vi "Get Worker Terminals.vi"(11 "Worker VI":refnum<vi>) -> (1 "Special Terminals":T1, 2 "Types":T2[](array[typedef]), 3 "Worker VI out":refnum<vi>)   [LabVIEW 2020, in "FlexBlock.xnode"]
uses:
  FlexBlock.xnode
  FlexBlocks/Type Descriptor.ctl
  FlexBlocks/Terminal Direction.ctl
  FlexBlocks/Value Mode.ctl
  FlexBlocks/Terminal State.ctl
  FlexBlocks/Special Terminal.ctl
  FlexBlocks/Special Terminal Indices.ctl
  FlexBlocks/Worker Action.ctl
  FlexBlocks/FlexBlocks.lvlib
  <vilib>/Utility/Data Type/NI_Data Type.lvlib
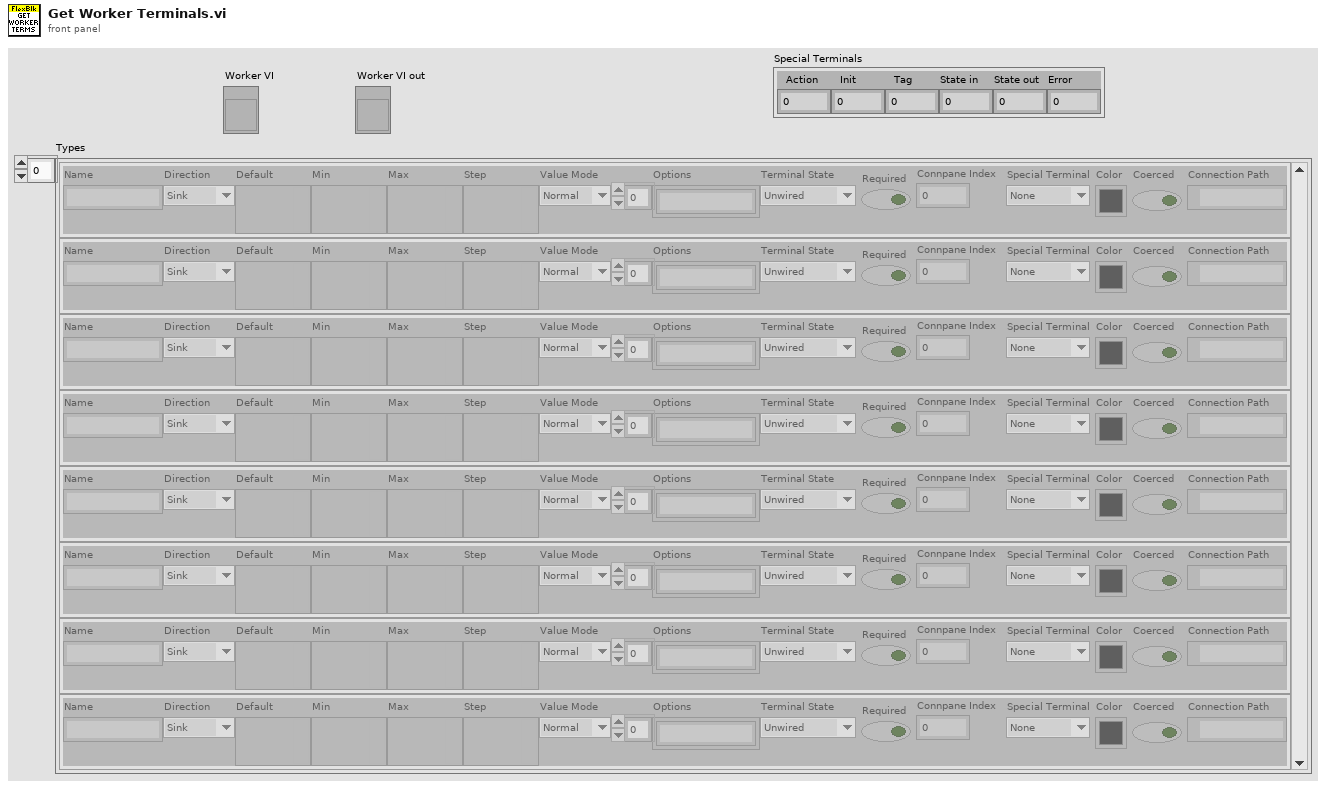
[diagram p1: front panel]
types:
  T1 = typedef "FlexBlocks.lvlib/Special Terminal Indices.ctl" = cluster{"Action":i32, "Init":i32, "Tag":i32, "State in":i32, "State out":i32, "Error":i32}
  T2 = typedef "FlexBlocks.lvlib/Type Descriptor.ctl" = cluster{"Name":string, "Direction":T3, "Default":variant, "Min":variant, "Max":variant, "Step":variant, "Value Mode":T4, "Options":string[], "Terminal State":T5, "Required":bool, "Connpane Index":i32, "Special Terminal":T6, "Color":u32, "Coerced":bool, "Connection Path":path}
  T3 = typedef "FlexBlocks.lvlib/Terminal Direction.ctl" = enum16{"Sink", "Source"}
  T4 = typedef "FlexBlocks.lvlib/Value Mode.ctl" = enum16{"Normal", "Range", "Select"}
  T5 = typedef "FlexBlocks.lvlib/Terminal State.ctl" = enum16{"Unwired", "BadType", "BadRef", "Channel", "Value", "Control Ref"}
  T6 = typedef "FlexBlocks.lvlib/Special Terminal.ctl" = enum16{"None", "Action", "Init", "Tag", "State in", "State out", "Error"}
  T7 = typedef "FlexBlocks.lvlib/Worker Action.ctl" = enum16{"Start", "Work", "Stop"}
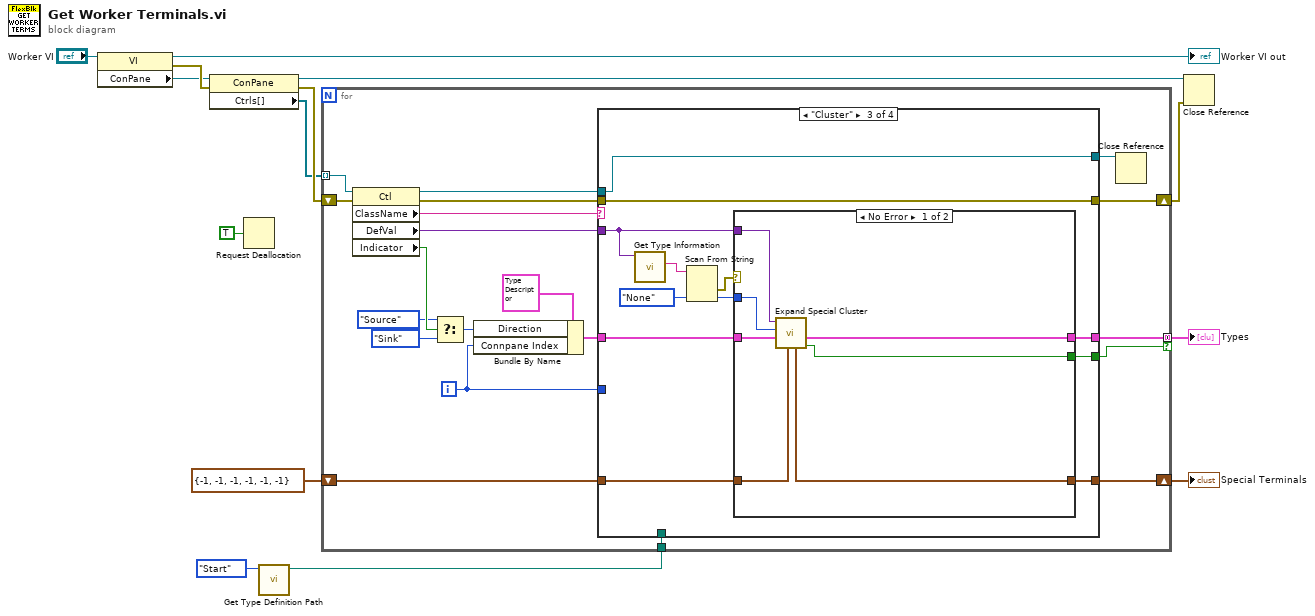
[diagram p0: block diagram]
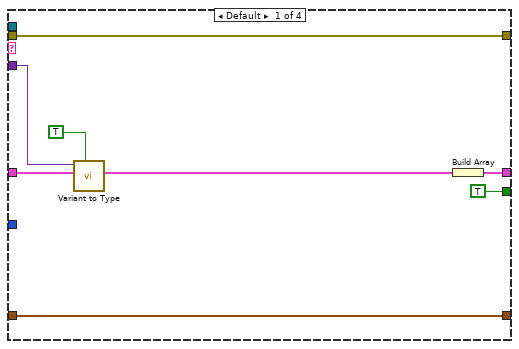
[diagram p2: hidden frame]
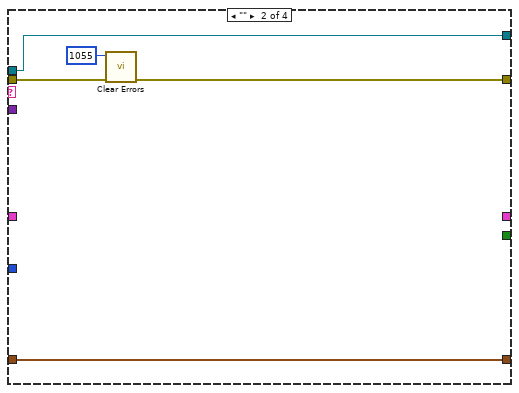
[diagram p3: hidden frame]
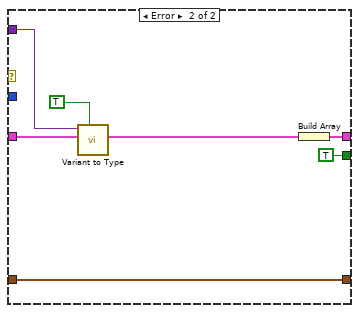
[diagram p4: hidden frame]
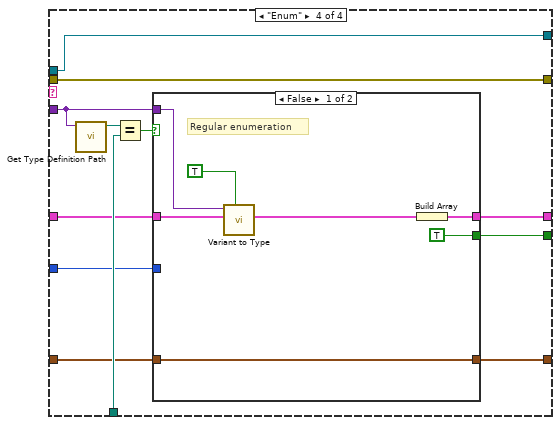
[diagram p5: hidden frame]
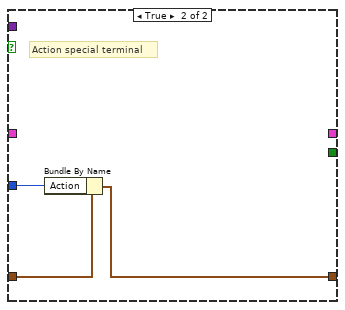
[diagram p6: hidden frame]
diagram:
  n1 = property class="VI"(reference="Worker VI") -> (reference out=→"Worker VI out":refnum<vi>, error out=w13:errorcluster, "ConPane"=w12:refnum<vi>)  [unwired: 1 in]
  n2 = property class="ConPane"(reference=w12, error in=w13) -> (reference out=w7:refnum<vi>, error out=w14:errorcluster, "Ctrls[]"=w9:refnum<vi>[])
  n3 = Request Deallocation(TRUE ("flag")) -> ()
  n4 = call <vilib>:"Get Type Definition Path.vi"("variant"=Worker_Action."Start" ("Action")) -> ("type definition path"=w3:path)  [unwired: 9 in, 1 out]
  n5 = for {
    tunnel: w9 -> [w33] mode=indexing
    shift-right: [w32] -> w6
    shift-left: w14 -> [w34]
    tunnel: w3 -> [w22]
    shift-right: [w19] -> w2
    shift-left: T1 {"Action"=-1, "Init"=-1, "Tag"=-1, "State in"=-1, "State out"=-1, "Error"=-1} ("Special Term Indices") -> [w21]
    tunnel: [w18] -> w1 mode=concatenating if=w17
    i -> [w15]
    n6 = property class="Ctl"(reference=w33, error in=w34) -> (reference out=w30:refnum<vi>, error out=w29:errorcluster, "ClassName"=w31:string, "DefVal"=w16:variant, "Indicator"=w27:bool)
    n7 = Select(t=Terminal_Direction."Source" ("Direction"), s=w27, f=Terminal_Direction."Sink" ("Direction")) -> (s? t:f=w26:T3)
    n8 = Bundle By Name(cluster=T2 {"Name"="", "Direction"=enum."Sink", "Default"=variant, "Min"=variant, "Max"=variant, "Step"=variant, "Value Mode"=enum."Normal", "Options"=[], "Terminal State"=enum."Unwired", "Required"=FALSE, "Connpane Index"=0, "Special Terminal"=enum."None", "Color"=0, "Coerced"=FALSE, "Connection Path"=path ""} ("Type Descriptor"), "Direction"=w26, "Connpane Index"=w15) -> (w23:T2)
    n9 = case shown="\"Cluster\"" w31 {
      tunnel: [w39 w47 w50 w82] -> w32
      tunnel: w30 -> [_ w43 w51 w81]
      tunnel: w29 -> [w39 w44 w50 w82]
      tunnel: w23 -> [w38 _ w53 w77]
      tunnel: w16 -> [w37 _ w52 w75]
      tunnel: w22 -> [_ _ _ w84]
      tunnel: w21 -> [w42 w45 w56 w80]
      tunnel: w15 -> [_ _ _ w79]
      tunnel: [_ w43 w51 w81] -> w20
      tunnel: [w42 w45 w55 w78] -> w19
      tunnel: [w40 _ w49 w74] -> w18
      tunnel: [TRUE ("Save Types?") _ w48 w76] -> w17
      frame Default {
        n10 = call "Variant to Type.vi"("Required? (F)"=TRUE ("Required"), "Type In"=w38, "Value"=w37) -> ("Type"=w36:T2)  [unwired: 8 in]
        n11 = Build Array(w36) -> (w40:T2[])
      }
      frame "" {
        n12 = call <vilib>:"Clear Errors.vi"("error in (no error)"=w44, "specific error code to clear (0: all)"=1055) -> ("error out"=w47:errorcluster)  [unwired: 4 in, 1 out]
      }
      frame "Cluster" {
        n13 = call <vilib>:"Get Type Information.vi"("variant"=w52) -> ("name"=w59:string)  [unwired: 6 in, 4 out]
        n14 = Scan From String(input string=w59, default 1=Special_Terminal."None" ("Special Terminal")) -> (error out=w54:errorcluster, output 1=w57:T6)  [unwired: 3 in, 2 out]
        n15 = case shown="No Error" w54 {
          tunnel: w57 -> [w64 _]
          tunnel: w56 -> [w61 w72]
          tunnel: [w60 w72] -> w55
          tunnel: w53 -> [w66 w70]
          tunnel: w52 -> [w65 w71]
          tunnel: [w62 w68] -> w49
          tunnel: [w63 TRUE ("Save Types?")] -> w48
          frame No Error {
            n16 = call "Expand Special Cluster.vi"("Special Term Indices In"=w61, "Initial Type Descriptor"=w66, "Special Terminal"=w64, "Variant"=w65) -> ("Save Types?"=w63:bool, "Contained Types"=w62:T2[], "Special Term Indices"=w60:T1)  [unwired: 5 in]
          }
          frame Error {
            n17 = call "Variant to Type.vi"("Required? (F)"=TRUE ("Required"), "Type In"=w70, "Value"=w71) -> ("Type"=w69:T2)  [unwired: 8 in]
            n18 = Build Array(w69) -> (w68:T2[])
          }
        }
      }
      frame "Enum" {
        n19 = call <vilib>:"Get Type Definition Path.vi"("variant"=w75) -> ("type definition path"=w85:path)  [unwired: 9 in, 1 out]
        n20 = Equal?(x=w85, y=w84) -> (x = y?=w83:bool)
        n21 = case shown="False" w83 {
          tunnel: w80 -> [w92 w95]
          tunnel: w79 -> [_ w94]
          tunnel: [w92 w93] -> w78
          tunnel: w77 -> [w89 _]
          tunnel: [TRUE _] -> w76
          tunnel: w75 -> [w88 _]
          tunnel: [w90 _] -> w74
          frame False {
            # "Regular enumeration"
            n22 = call "Variant to Type.vi"("Required? (F)"=TRUE ("Required"), "Type In"=w89, "Value"=w88) -> ("Type"=w86:T2)  [unwired: 8 in]
            n23 = Build Array(w86) -> (w90:T2[])
          }
          frame True {
            # "Action special terminal"
            n24 = Bundle By Name(cluster=w95, "Action"=w94) -> (w93:T1)
          }
        }
      }
    }
    n25 = Close Reference(reference=w20) -> ()  [unwired: 1 in, 1 out]
  }
  "Types" <- w1
  "Special Terminals" <- w2
  n26 = Close Reference(reference=w7, error in (no error)=w6) -> ()  [unwired: 1 out]
